vi "Create.vi"(8 "error in (no error)":errorcluster, 11 "group count (1)":u64=1) -> (0 "error out":errorcluster, 3 "Transfer Group Status":refnum<class "Transfer Group Status.lvclass">)   [LabVIEW 2017, in "DSF Core.lvlib" / "Transfer Group Status.lvclass"]
uses:
  Transfer Group Status.lvclass
  C:/Program Files (x86)/National Instruments/LabVIEW 2017/vi.lib/NI/Memory Manager/Classes/Pointer/Pointer.lvclass
  DSF Configuration API/Public/Controls/DSF Transfer Group Status.ctl
  <vilib>/NI/Memory Manager/Classes/Pointer/Pointer.lvclass/Pointer.ctl
  9fcae784-2296-4031-aa96-aa7f3b317fc3.vi
  f2b94dab-149e-4a40-9225-6eb4de63dfa7.vi
  9fcae784-2296-4031-aa96-aa7f3b317fc3.vi/5a7c06e1-78d0-476c-bb75-dd61e1c5940c.vi
  <vilib>/NI/Memory Manager/Classes/Pointer/Allocate.vi
  f2b94dab-149e-4a40-9225-6eb4de63dfa7.vi/e92f1dc3-74c9-4aec-9255-c3559d55296b.vi
  <vilib>/NI/Memory Manager/Classes/Pointer/Get Address.vi
  <vilib>/NI/Memory Manager/Classes/Pointer/Check Size (0D).vi
  <vilib>/NI/Memory Manager/Classes/Pointer/Set Address.vi
  <vilib>/NI/Memory Manager/Classes/Pointer/Set Size.vi
  <vilib>/NI/Memory Manager/Classes/Pointer/Set Internal.vi
  <vilib>/NI/Memory Manager/Classes/Pointer/Errors.vi
  <vilib>/NI/Memory Manager/Classes/Pointer/Out of Bounds.vi
  <vilib>/NI/Memory Manager/Classes/Pointer/Get Size.vi
  <vilib>/NI/Memory Manager/VIs/Source.Write.String.vi
  <vilib>/NI/Memory Manager/Classes/Pointer/Write Pointer Size.vi
  <vilib>/NI/Memory Manager/Classes/Pointer/Create Error.vi
  <vilib>/NI/Memory Manager/VIs/Source.Write.Scalar.Base10.vi
  <vilib>/NI/Memory Manager/VIs/Source.Write.Scalar.Base10 (U64).vi
  <vilib>/NI/Memory Manager/VIs/New Error Cluster Constant.vi
  <vilib>/NI/Memory Manager/VIs/New Error Cluster Constant (512B).vi
  <vilib>/NI/Memory Manager/VIs/Error Cluster.Set Status.vi
  <vilib>/NI/Memory Manager/VIs/Error Cluster.Set Code.vi
  <vilib>/NI/Memory Manager/VIs/Error Cluster.Set VI Source.vi
  <vilib>/NI/Memory Manager/Constants/Constants.vi
  <vilib>/NI/Memory Manager/Constants/Library Name.vi
  <vilib>/NI/Memory Manager/Classes/Pointer/Pointer Error Info.vi
  <vilib>/NI/Memory Manager/Constants/Pointer Class Name.vi
  DSF Core.lvlib
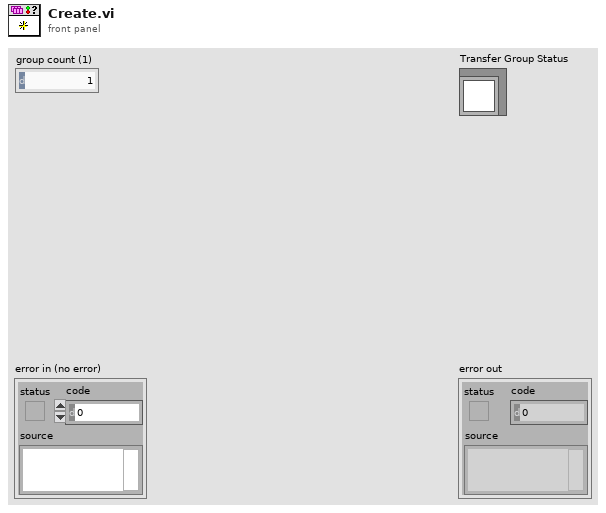
[diagram p1: front panel]
types:
  T1 = typedef "DSF Core.lvlib/DSF Transfer Group Status.ctl" = cluster{"late count":u64, "iteration":u64}
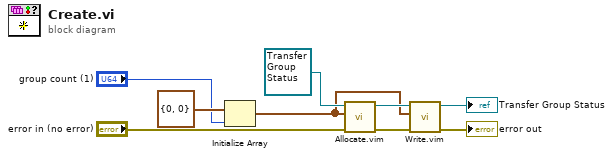
[diagram p0: block diagram]
diagram:
  n1 = Initialize Array(T1 {"late count"=0, "iteration"=0} ("Transfer Group status"), "group count (1)") -> (w2:T1[])
  n2 = call "Allocate.vim"("error in (no error)"="error in (no error)", "anything"=w2, "Pointer in"=refnum<class "Transfer Group Status.lvclass"> refnum ("Transfer Group Status in")) -> ("error out"=w6:errorcluster, "Pointer out"=w7:refnum<class "Transfer Group Status.lvclass">)  [unwired: 7 in]
  n3 = call "Write.vim"("error in (no error)"=w6, "buffer in"=w2, "Pointer in"=w7) -> ("error out"=→"error out":errorcluster, "Pointer out"=→"Transfer Group Status":refnum<class "Transfer Group Status.lvclass">)  [unwired: 6 in, 1 out]
